vi "Stop DAQ.vi"(8 "error in (no error)":errorcluster, 11 "Application Manager in":refnum<class "Application Manager.lvclass">) -> (0 "error out":errorcluster, 3 "Application Manager out":refnum<class "Application Manager.lvclass">)   [LabVIEW 2025, in "Application Manager.lvlib" / "Application Manager.lvclass"]
uses:
  Application Manager.lvclass
  Application Manager.lvclass/Application Manager.ctl
  <vilib>/ActorFramework/Message Enqueuer/Message Enqueuer.lvclass/Message Enqueuer.ctl
  <vilib>/ActorFramework/Message Enqueuer/Enqueue.vi
  DAQ Interface/DAQ Interface Messages/Stop DAQ Msg/Stop DAQ Msg.lvclass
  <vilib>/ActorFramework/Message Priority Queue/Priority Enqueue.vi
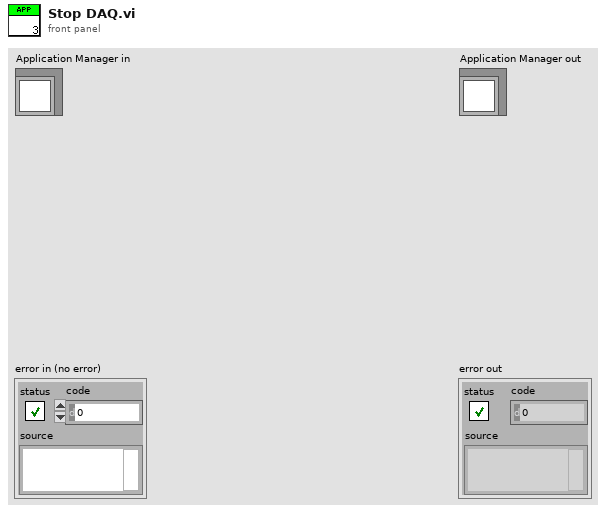
[diagram p1: front panel]
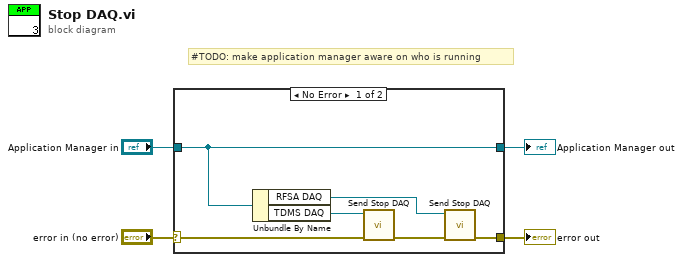
[diagram p0: block diagram]
diagram:
  # "#TODO: make application manager aware on who is running"
  n1 = case shown="No Error" "error in (no error)" {
    selector: "error in (no error)" -> [w8 w12]
    tunnel: [w7 w12] -> w3
    tunnel: [w10 w11] -> w1
    tunnel: "Application Manager in" -> [w10 w11]
    frame No Error {
      n2 = Unbundle By Name(w10) -> ("RFSA DAQ"=w5:refnum<class "Message Enqueuer.lvclass">, "TDMS DAQ"=w9:refnum<class "Message Enqueuer.lvclass">)
      n3 = call "Send Stop DAQ.vi"("error in (no error)"=w8, "Message Enqueuer"=w9) -> ("error out"=w6:errorcluster)  [unwired: 8 in, 1 out]
      n4 = call "Send Stop DAQ.vi"("error in (no error)"=w6, "Message Enqueuer"=w5) -> ("error out"=w7:errorcluster)  [unwired: 8 in, 1 out]
    }
    frame Error {
    }
  }
  "error out" <- w3
  "Application Manager out" <- w1
